vi "Test User Interface API.vi"() -> ()   [LabVIEW 2020]
doc: "User Interface API Tester."
uses:
  User Interface.lvlib
panel:
  in  "Show Block Diagram":bool
  in  "Stop Module":bool
  in  "Start Module":bool
  in  "Hide Module Panel":bool
  in  "Show Module Panel":bool
  out "Status":string
  out "Module Running?":bool
  # "This VI tests the API for the Module."
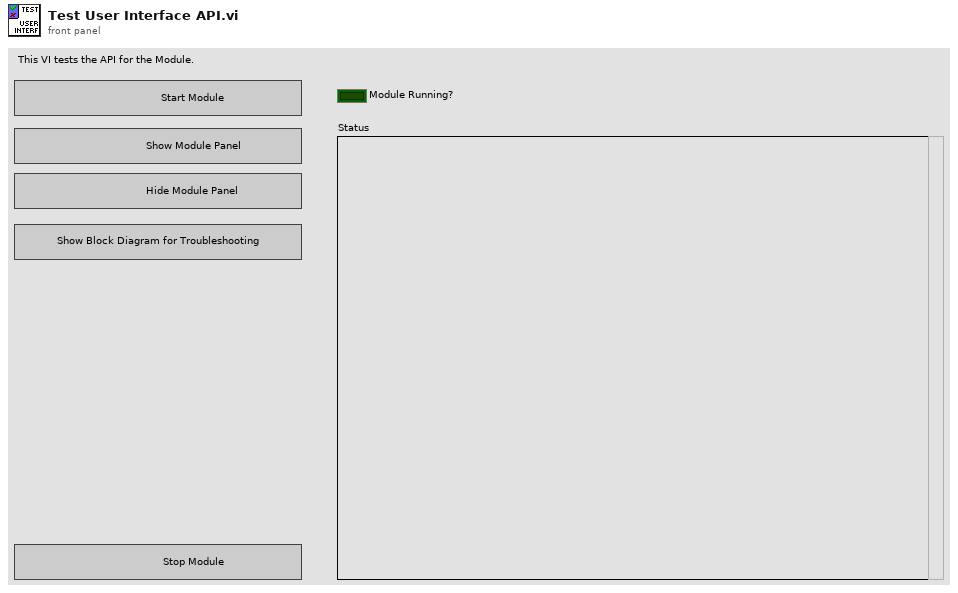
[diagram p1: front panel]
types:
  T1 = typedef "User Interface.lvlib/Broadcast Events--cluster.ctl" = cluster{"Module Did Init":refnum<user-event>, "Status Updated":refnum<user-event>, "Error Reported":refnum<user-event>, "Did Something":refnum<user-event>, "Module Did Stop":refnum<user-event>, "Update Module Execution Status":refnum<user-event>}
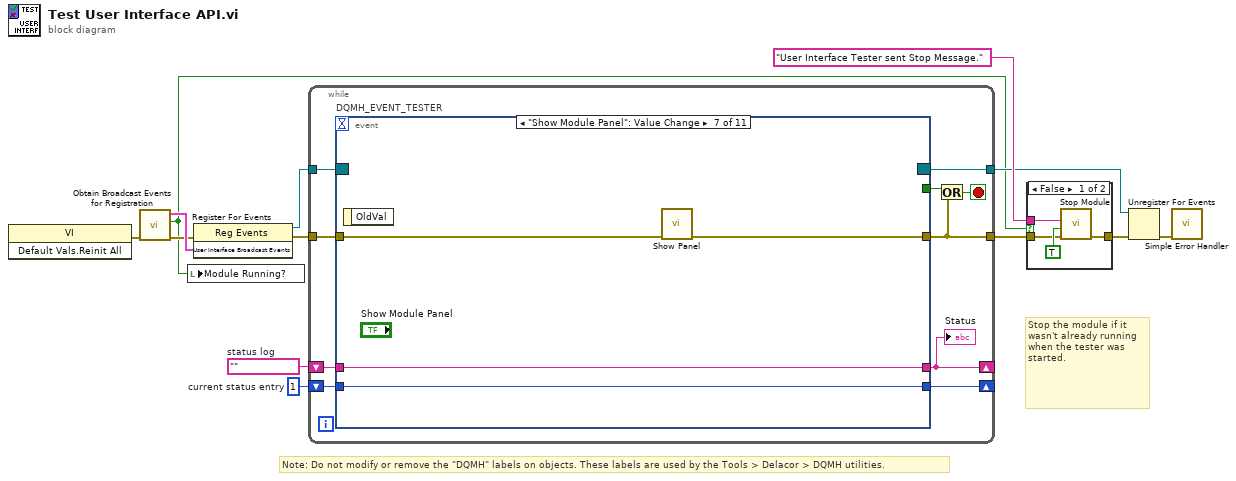
[diagram p0: block diagram]
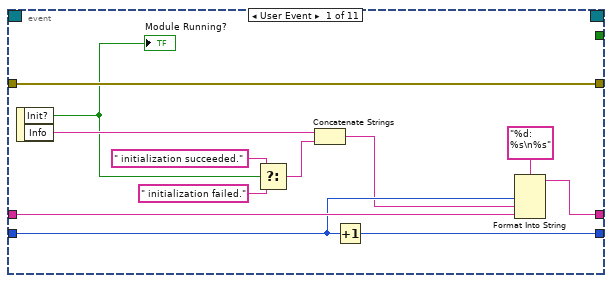
[diagram p3: hidden frame]
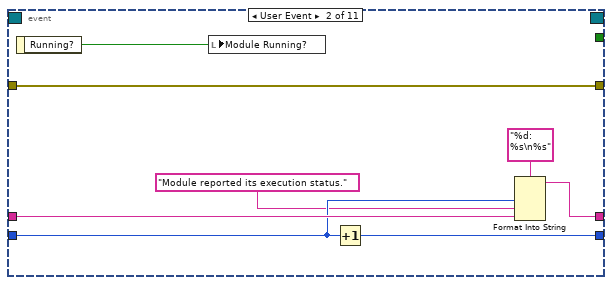
[diagram p4: hidden frame]
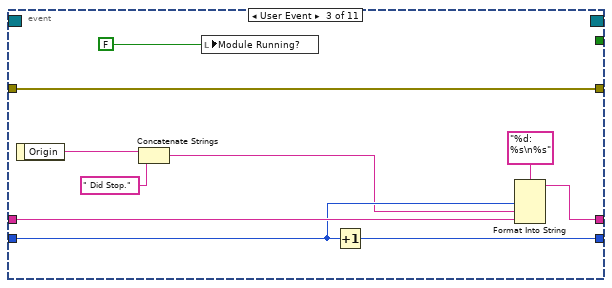
[diagram p5: hidden frame]
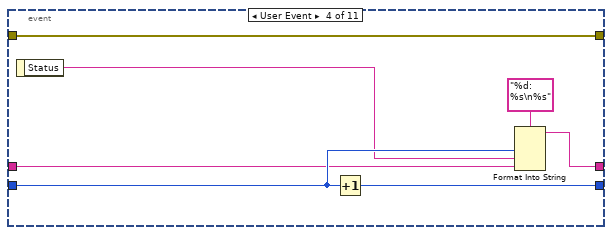
[diagram p6: hidden frame]
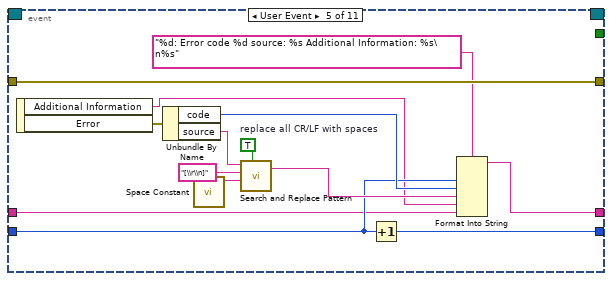
[diagram p7: hidden frame]
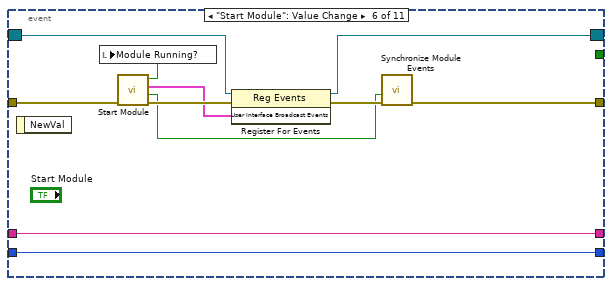
[diagram p8: hidden frame]
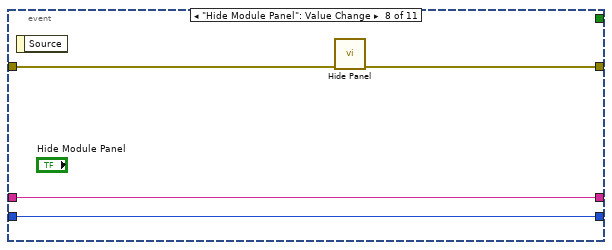
[diagram p9: hidden frame]
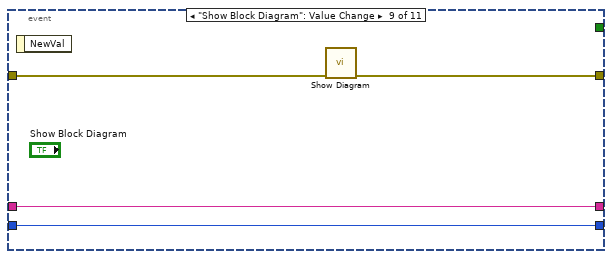
[diagram p10: hidden frame]
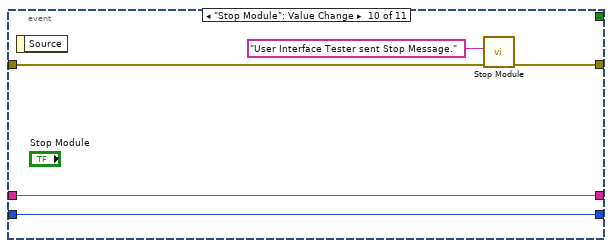
[diagram p11: hidden frame]
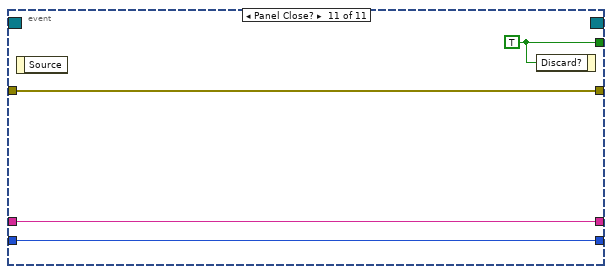
[diagram p12: hidden frame]
diagram:
  w10 = 1  # current status entry
  w11 = ""  # status log
  # "Stop the module if it wasn't already running when the tester was started."
  # "Note: Do not modify or remove the \"DQMH\" labels on objects. These labels are used by the Tools > Delacor > DQMH utilities."
  n1 = invoke class="VI" method="Default Vals.Reinit All"() -> (error out=w5:errorcluster)  [unwired: 3 in, 2 out]
  n2 = call "Obtain Broadcast Events for Registration.vi"("error in (no error)"=w5) -> ("error out"=w4:errorcluster, "Already running?"=w3:bool, "User Interface Broadcast Events"=w8:T1)  [unwired: 8 in]
  n3 = local write "Module Running?"(w3) -> ()
  n4 = register-events(error in=w4, w8) -> (reference out=w7:refnum<event-registration>, error out=w9:errorcluster)  [unwired: 1 in]
  n5 = while {
    tunnel: w7 -> [w23]
    tunnel: [w14] -> w2
    shift-right: [w18] -> _
    shift-left: w11 -> [w20]
    shift-right: [w19] -> _
    shift-left: w10 -> [w21]
    tunnel: w9 -> [w16]
    tunnel: [w15] -> w6
    stop <- w17 stop-if-true
    n6 = event "DQMH_EVENT_TESTER" shown="[6] \"Show Module Panel\": Value Change" {
      selector: w23 -> [_ _ _ _ _ w79 _ _ _ _ _]
      dyn-events: [_ _ _ _ _ w78 _ _ _ _ _] -> w15
      timeout: _ -> [_ _ _ _ _ _ _ _ _ _ _]
      tunnel: [_ _ _ _ _ _ _ _ _ _ w106] -> w22
      tunnel: [w35 w37 w44 w54 w74 w77 w89 w93 w94 w100 w103] -> w14
      tunnel: w21 -> [w32 w41 w51 w57 w64 w82 w87 w91 w95 w101 w104]
      tunnel: w20 -> [w33 w42 w52 w56 w62 w83 w88 w92 w96 w102 w105]
      tunnel: [w30 w39 w49 w58 w65 w83 w88 w92 w96 w102 w105] -> w18
      tunnel: [w31 w40 w50 w60 w63 w82 w87 w91 w95 w101 w104] -> w19
      tunnel: w16 -> [w35 w37 w44 w54 w74 w76 w86 w90 w97 w98 w103]
      event User Event {
        n7 = event-data() -> ("Init?"=w27:bool, "Info"=w29:string)  [unwired: 1 in]
        "Module Running?" <- w27
        n8 = Select(t=" initialization succeeded.", s=w27, f=" initialization failed.") -> (s? t:f=w24:string)
        n9 = Concatenate Strings(w29, w24) -> (w28:string)
        n10 = Increment(x=w32) -> (x+1=w31:i32)
        n11 = Format Into String(format string="%d: %s\n%s", w32, w28, w33) -> (resulting string=w30:string)  [unwired: 2 in, 1 out]
      }
      event User Event {
        n12 = event-data() -> ("Running?"=w36:bool)  [unwired: 1 in]
        n13 = local write "Module Running?"(w36) -> ()
        n14 = Increment(x=w41) -> (x+1=w40:i32)
        n15 = Format Into String(format string="%d: %s\n%s", w41, "Module reported its execution status.", w42) -> (resulting string=w39:string)  [unwired: 2 in, 1 out]
      }
      event User Event {
        n16 = event-data() -> ("Origin"=w48:string)  [unwired: 1 in]
        n17 = Concatenate Strings(w48, " Did Stop.") -> (w47:string)
        n18 = local write "Module Running?"(FALSE ("Module Did Init?")) -> ()
        n19 = Increment(x=w51) -> (x+1=w50:i32)
        n20 = Format Into String(format string="%d: %s\n%s", w51, w47, w52) -> (resulting string=w49:string)  [unwired: 2 in, 1 out]
      }
      event User Event {
        n21 = event-data() -> ("Status"=w55:string)  [unwired: 1 in]
        n22 = Increment(x=w57) -> (x+1=w60:i32)
        n23 = Format Into String(format string="%d: %s\n%s", w57, w55, w56) -> (resulting string=w58:string)  [unwired: 2 in, 1 out]
      }
      event User Event {
        w70 = TRUE  # replace all CR/LF with spaces
        n24 = event-data() -> ("Additional Information"=w61:string, "Error"=w66:errorcluster)  [unwired: 1 in]
        n25 = Unbundle By Name(w66) -> ("code"=w67:i32, "source"=w68:string)
        n26 = call <vilib>:"Space Constant.vi"() -> ("String"=w71:string)
        n27 = call <vilib>:"Search and Replace Pattern.vi"("string"=w68, "regular expression (\"\")"="[\\r\\n]" ("regular expression (\"\")"), "replace string (\"\")"=w71, "replace all? (F)"=w70) -> ("result string"=w69:string)  [unwired: 1 in, 1 out]
        n28 = Increment(x=w64) -> (x+1=w63:i32)
        n29 = Format Into String(format string="%d: Error code %d source: %s Additional Information: %s\n%s", w64, w67, w69, w61, w62) -> (resulting string=w65:string)  [unwired: 2 in, 1 out]
      }
      event "Start Module": Value Change {
        n30 = event-data() -> ()  [unwired: 1 in, 1 out]
        n31 = call "Start Module.vi"("error in (no error)"=w76) -> ("error out"=w84:errorcluster, "Wait for Event Sync?"=w81:bool, "User Interface Broadcast Events"=w80:T1, "Module Was Already Running?"=w75:bool)  [unwired: 7 in]
        n32 = local write "Module Running?"(w75) -> ()
        n33 = register-events(reference=w79, error in=w84, w80) -> (reference out=w78:refnum<event-registration>, error out=w85:errorcluster)
        n34 = call "Synchronize Module Events.vi"("error in"=w85, "Wait for Event Sync?"=w81) -> ("error out"=w77:errorcluster)  [unwired: 9 in]
      }
      event "Show Module Panel": Value Change {
        n35 = event-data() -> ()  [unwired: 1 in, 1 out]
        n36 = call "Show Panel.vi"("error in (no error)"=w86) -> ("error out"=w89:errorcluster)  [unwired: 10 in]
      }
      event "Hide Module Panel": Value Change {
        n37 = event-data() -> ()  [unwired: 1 in, 1 out]
        n38 = call "Hide Panel.vi"("error in (no error)"=w90) -> ("error out"=w93:errorcluster)  [unwired: 10 in]
      }
      event "Show Block Diagram": Value Change {
        n39 = event-data() -> ()  [unwired: 1 in, 1 out]
        n40 = call "Show Diagram.vi"("error in (no error)"=w97) -> ("error out"=w94:errorcluster)  [unwired: 10 in]
      }
      event "Stop Module": Value Change {
        n41 = event-data() -> ()  [unwired: 1 in, 1 out]
        n42 = call "Stop Module.vi"("error in"=w98, "Origin"="User Interface Tester sent Stop Message.") -> ("error out"=w100:errorcluster)  [unwired: 9 in]
      }
      event Panel Close? {
        w106 = TRUE ("Discard?")
        n43 = event-data() -> ()  [unwired: 1 in, 1 out]
        n44 = event-data("Discard?"=w106) -> ()  [unwired: 1 in, 1 out]
      }
    }
    "Status" <- w18
    n45 = Or(x=w22, y=w14) -> (x .or. y?=w17:bool)
  }
  n46 = case shown="False" w3 {
    tunnel: [w110 w111] -> w13
    tunnel: "User Interface Tester sent Stop Message." ("Origin") -> [w109 _]
    tunnel: w2 -> [w107 w111]
    frame False {
      n47 = call "Stop Module.vi"("error in"=w107, "Wait for Module to Stop? (F)"=TRUE ("Wait for Module to stop?"), "Origin"=w109) -> ("error out"=w110:errorcluster)  [unwired: 8 in]
    }
    frame True {
    }
  }
  n48 = Unregister For Events(event registration refnum=w6, error in=w13) -> (error out=w1:errorcluster)
  n49 = call <vilib>:"Simple Error Handler.vi"("error in (no error)"=w1) -> ()  [unwired: 4 in, 5 out]
